vi "ConfigureSensorType.vi"(0 "axis in":cluster{"keyHandle":u32, "nodeId":u16}={"keyHandle"=0, "nodeId"=1}, 1 "SensorType":u16(ring) items=["Unknown sensor", "Incremental encoder with index (3-channel)", "Incremental encoder without index (2-channel)", "Hall sensors", "SSI absolute encoder - binary coded data", "SSI absolute encoder - grey coded data", "Incremental encoder 2 with index (3-channel)", "Incremental encoder 2 without index (2-channel)", "Absolute incremental encoder with index (3-channel)", "Absolute incremental encoder with index (2-channel)"], 2 "incremental encoder configuration":T2, 3 "hallsensor configuration":cluster{"invertedPolarity":i32}, 4 "SSI encoder configuration":T1, 5 "error in (no error)":errorcluster) -> (14 "axis out":cluster{"keyHandle":u32, "nodeId":u16}={"keyHandle"=0, "nodeId"=1}, 19 "error out":errorcluster)   [LabVIEW 2017, in "maxonEPOS.lvlib"]
doc: "<B>ConfigureSensorType</B> writes the correct sensor type to the device. Parameters from the sensor type can be set."
uses:
  Examples/maxonEPOS.lvlib
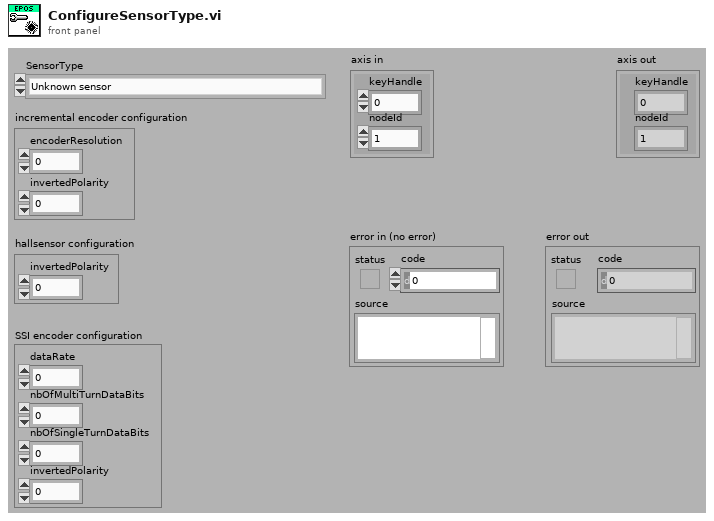
[diagram p1: front panel]
types:
  T1 = cluster{"dataRate":u16, "nbOfMultiTurnDataBits":u16, "nbOfSingleTurnDataBits":u16, "invertedPolarity":i32}
  T2 = cluster{"encoderResolution":u32, "invertedPolarity":i32}
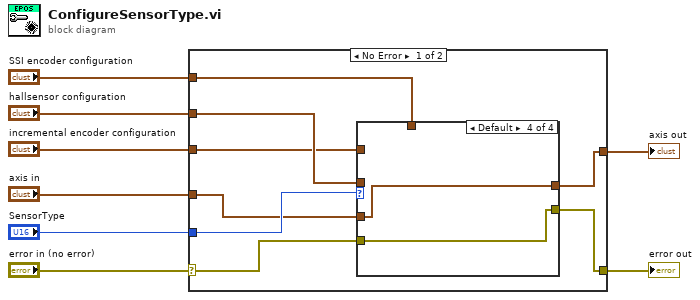
[diagram p0: block diagram]
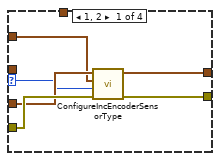
[diagram p2: hidden frame]
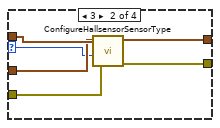
[diagram p3: hidden frame]
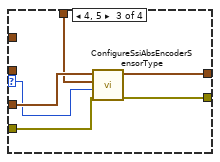
[diagram p4: hidden frame]
diagram:
  n1 = case shown="No Error" "error in (no error)" {
    selector: "error in (no error)" -> [w10 w38]
    tunnel: [w15 w38] -> w7
    tunnel: [w14 w37] -> w6
    tunnel: "axis in" -> [w9 w37]
    tunnel: "SensorType" -> [w16 _]
    tunnel: "incremental encoder configuration" -> [w11 _]
    tunnel: "hallsensor configuration" -> [w12 _]
    tunnel: "SSI encoder configuration" -> [w13 _]
    frame No Error {
      n2 = case shown="Default" w16 {
        selector: w16 -> [w17 w23 w29 _]
        tunnel: w10 -> [w20 w26 w34 w35]
        tunnel: [w21 w25 w33 w35] -> w15
        tunnel: [w22 w24 w32 w36] -> w14
        tunnel: w9 -> [w19 w27 w31 w36]
        tunnel: w13 -> [_ _ w30 _]
        tunnel: w12 -> [_ w28 _ _]
        tunnel: w11 -> [w18 _ _ _]
        frame 1, 2 {
          n3 = call "ConfigureIncEncoderSensorType.vi"("error in (no error)"=w20, "SensorType"=w17, "incremental encoder configuration"=w18, "axis in"=w19) -> ("error out"=w21:errorcluster, "axis out"=w22:cluster{"keyHandle":u32, "nodeId":u16})  [unwired: 2 in]
        }
        frame 3 {
          n4 = call "ConfigureHallsensorSensorType.vi"("error in (no error)"=w26, "SensorType"=w23, "hallsensor configuration"=w28, "axis in"=w27) -> ("error out"=w25:errorcluster, "axis out"=w24:cluster{"keyHandle":u32, "nodeId":u16})  [unwired: 2 in]
        }
        frame 4, 5 {
          n5 = call "ConfigureSsiAbsEncoderSensorType.vi"("error in (no error)"=w34, "SensorType"=w29, "SSI encoder configuration"=w30, "axis in"=w31) -> ("error out"=w33:errorcluster, "axis out"=w32:cluster{"keyHandle":u32, "nodeId":u16})  [unwired: 2 in]
        }
        frame Default {
        }
      }
    }
    frame Error {
    }
  }
  "error out" <- w7
  "axis out" <- w6
